vi "DSF.Engine.Plugin.Parse Transfer Group.vi"(8 "error in (no error)":errorcluster, 10 "Transfer Group in":refnum<class "DSF.Engine.Transfer Group.lvclass">, 11 "Plugin in":refnum<class "Plugin.lvclass">) -> (0 "error out":errorcluster, 2 "Transfer Group out":refnum<class "DSF.Engine.Transfer Group.lvclass">, 3 "Plugin out":refnum<class "Plugin.lvclass">)   [LabVIEW 2016, in "DSF.Engine.lvlib" / "Plugin.lvclass"]
uses:
  Plugin.lvclass
  Transfer/DSF.Engine.Transfer Group.lvclass
  Builder/DSF.Engine.Builder.lvclass
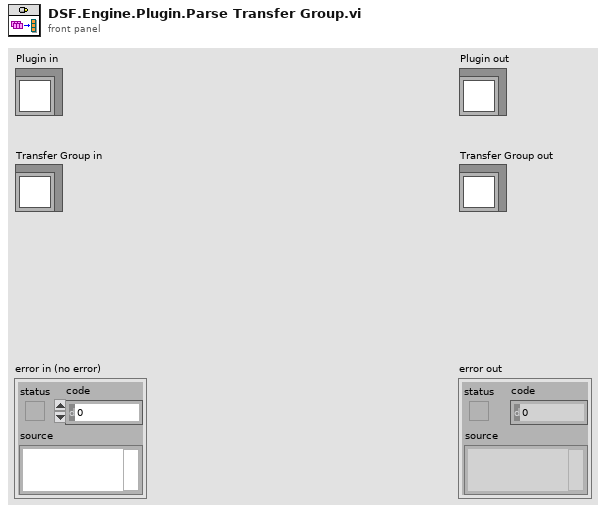
[diagram p1: front panel]
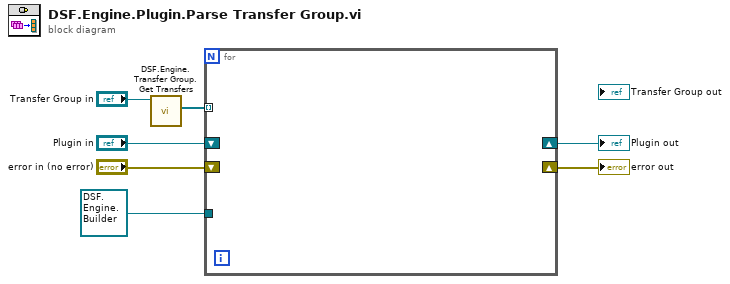
[diagram p0: block diagram]
diagram:
  n1 = call "DSF.Engine.Transfer Group.Get Transfers.vi"("Transfer Group in"="Transfer Group in") -> ("Transfers"=w4:refnum<class "DSF.Engine.Transfer.lvclass">[])  [unwired: 9 in, 1 out]
  n2 = for {
    tunnel: w4 -> [_] mode=indexing
    tunnel: refnum<class "DSF.Engine.Builder.lvclass"> refnum ("DSF.Engine.lvlib:Builder") -> [_]
    shift-right: [_] -> w2
    shift-left: "Plugin in" -> [_]
    shift-right: [_] -> w1
    shift-left: "error in (no error)" -> [_]
  }
  "error out" <- w1
  "Plugin out" <- w2
